vi "SetTriggerMode.vi"(9 "Trigger":refnum<vi>, 10 "ExposureMode":refnum<k24>, 11 "Digital in":refnum<vi>) -> ()   [LabVIEW 2019]
uses:
  Dependencies/PVCamNET.dll
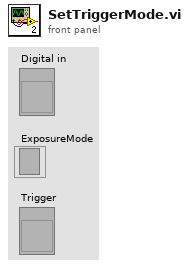
[diagram p1: front panel]
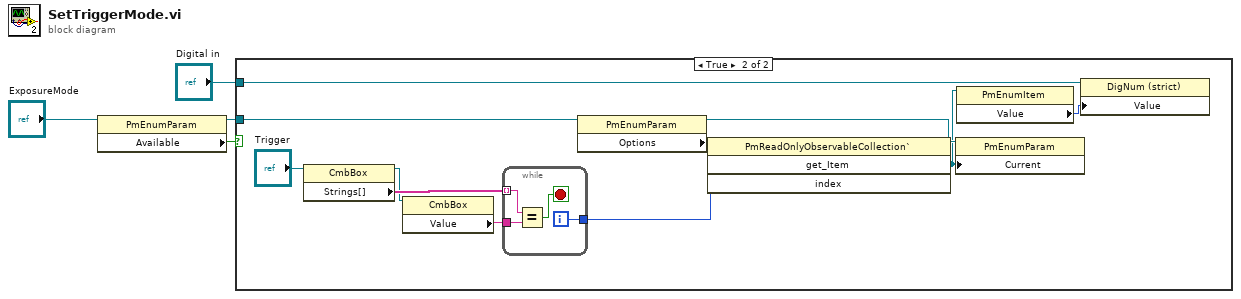
[diagram p0: block diagram]
diagram:
  n1 = property class="PmEnumParam"(reference="ExposureMode") -> (reference out=w3:refnum<k24>, "Available"=w2:bool)  [unwired: 1 in, 1 out]
  n2 = case shown="True" w2 {
    tunnel: w3 -> [_ w14]
    tunnel: "Digital in" -> [_ w8]
    frame False {
    }
    frame True {
      n3 = property class="CmbBox"(reference="Trigger") -> (reference out=w6:refnum<vi>, "Strings[]"=w15:string[])  [unwired: 1 in, 1 out]
      n4 = property class="CmbBox"(reference=w6) -> ("Value"=w5:string)  [unwired: 1 in, 2 out]
      n5 = while {
        tunnel: w15 -> [w19] mode=indexing
        tunnel: [w17] -> w12
        tunnel: w5 -> [w16]
        i -> [w17]
        stop <- w18 stop-if-true
        n6 = Equal?(x=w19, y=w16) -> (x = y?=w18:bool)
      }
      n7 = property class="PmEnumParam"(reference=w14) -> (reference out=w11:refnum<k24>, "Options"=w13:refnum<k24>)  [unwired: 1 in, 1 out]
      n8 = invoke class="PmReadOnlyObservableCollection`" method="get_Item"(reference=w13, "index"=w12) -> ("get_Item"=w10:refnum<k24>)  [unwired: 2 in, 3 out]
      n9 = property class="PmEnumParam"(reference=w11, "Current"=w10) -> ()  [unwired: 1 in, 2 out]
      n10 = property class="PmEnumItem"(reference=w10) -> ("Value"=w9:i32)  [unwired: 1 in, 2 out]
      n11 = property class="DigNum (strict)"(reference=w8, "Value"=w9) -> ()  [unwired: 1 in, 2 out]
    }
  }
